vi "AMC Create Message Queue.vi"(8 "error in (no error)":errorcluster, 9 "Initial Message Values":string[](array[string]), 10 "Initial Message Names":string[](array[string]), 11 "Message Queue Name":string) -> (0 "error out":errorcluster, 3 "Message Queue out":T1)   [LabVIEW 2017]
doc: "This VI creates a new local message queue or returns a reference to an existing message queue baseed on the queue name. You can pass in a list of initial messages which will be added to the queue."
uses:
  subVIs/TypeDefs/amc_Message Queue.ctl
  subVIs/TypeDefs/amc_Message.ctl
  Tools/Keyed Array/Tools_KeyedArray KeyedArray.ctl
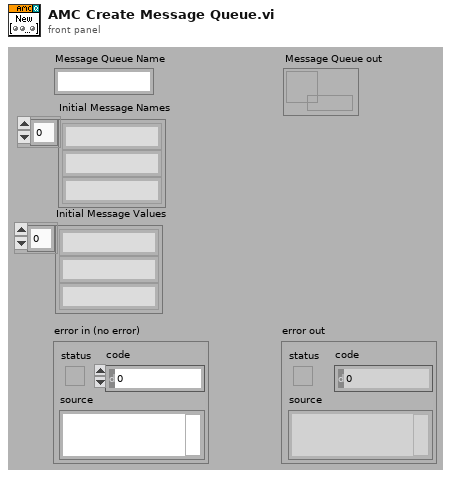
[diagram p1: front panel]
types:
  T1 = typedef "amc_Message Queue.ctl" = refnum<queue>
  T2 = typedef "amc_Message.ctl" = cluster{"Name":string, "Value":string, "Attributes":T3, "Receiver Host":string, "Receiver Process":string, "Source Host":string, "Source Process":string, "Priority Message":bool, "Acknowledge Message":bool}
  T3 = typedef "Tools_KeyedArray KeyedArray.ctl" = cluster{"keys":string[], "values":string[]}
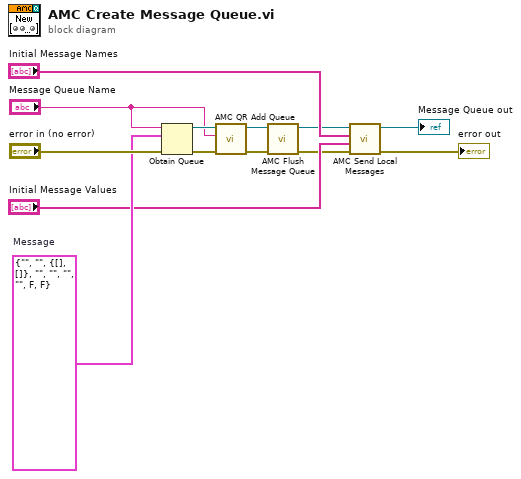
[diagram p0: block diagram]
diagram:
  w12 = T2 {"Name"="", "Value"="", "Attributes"={"keys"=[], "values"=[]}, "Receiver Host"="", "Receiver Process"="", "Source Host"="", "Source Process"="", "Priority Message"=FALSE, "Acknowledge Message"=FALSE}  # Message
  n1 = Obtain Queue(name (unnamed)="Message Queue Name", element data type=w12, error in (no error)="error in (no error)") -> (queue out=w6:refnum<queue>, error out=w7:errorcluster)  [unwired: 2 in, 1 out]
  n2 = call "AMC QR Add Queue .vi"("error in (no error)"=w7, "Name"="Message Queue Name", "Message Queue in"=w6) -> ("error out"=w4:errorcluster, "Message Queue out"=w3:T1)  [unwired: 7 out]
  n3 = call "AMC Flush Message Queue.vi"("error in (no error)"=w4, "Message Queue in"=w3) -> ("error out"=w1:errorcluster, "Message Queue out"=w2:T1)  [unwired: 7 out]
  n4 = call "AMC Send Local Messages.vi"("error in (no error)"=w1, "Message Values"="Initial Message Values", "Message Names"="Initial Message Names", "Message Queue in"=w2) -> ("error out"=→"error out":errorcluster, "Message Queue out"=→"Message Queue out":T1)  [unwired: 1 in, 5 out]
